vi "solar_voy_def Items Bit Offsets.vi"(10 "ITEMS in":T1[](array[typedef])) -> (1 "Bit Offsets":i32[](array[numeric]), 2 "ITEMS with Bit Offsets":T1[](array[typedef]))   [LabVIEW 2018]
doc: "This calculates the bit offsets for each item. If OFFSET is -1, this uses the current calculated bit offset."
uses:
  solar_voy_def_ctl ITEM TYPE.ctl
  type/solar_type Item Type.ctl
  solar_voy_def_ctl ITEM.ctl
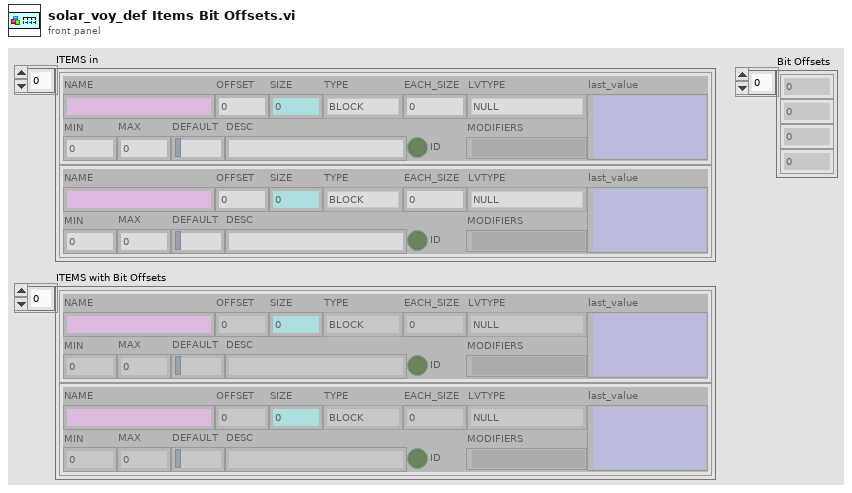
[diagram p1: front panel]
types:
  T1 = typedef "solar_voy_def_ctl ITEM.ctl" = cluster{"NAME":string, "OFFSET":i32, "SIZE":i32, "TYPE":T2, "EACH_SIZE":i32, "LVTYPE":T3, "MIN":dbl, "MAX":dbl, "DEFAULT":string, "DESC":string, "ID":bool, "MODIFIERS":variant, "last_value":variant}
  T2 = typedef "solar_voy_def_ctl ITEM TYPE.ctl" = enum8{"BLOCK", "INT", "UINT", "FLOAT", "STRING"}
  T3 = typedef "solar_type Item Type.ctl" = enum16{"NULL", "UNKNOWN", "CLUSTER", "I8", "I16", "I32", "I64", "U8", "U16", "U32", "U64", "U8_ENUM", "U16_ENUM", "U32_ENUM", "SGL", "DBL", "BOOLEAN", "STRING", "PATH", "VISA", "TAG", "TIME", "I8_1D", "I16_1D", "I32_1D", "I64_1D", "U8_1D", "U16_1D", "U32_1D", "U64_1D", "U8_ENUM_1D", "U16_ENUM_1D", "U32_ENUM_1D", "SGL_1D", "DBL_1D", "BOOLEAN_1D", "STRING_1D", "PATH_1D", "VISA_1D", "TAG_1D", "TIME_1D", "I8_2D", "I16_2D", "I32_2D", "I64_2D", "U8_2D", "U16_2D", "U32_2D", "U64_2D", "U8_ENUM_2D", "U16_ENUM_2D", "U32_ENUM_2D", "SGL_2D", "DBL_2D", "BOOLEAN_2D", "STRING_2D", "PATH_2D", "VISA_2D", "TAG_2D", "TIME_2D"}
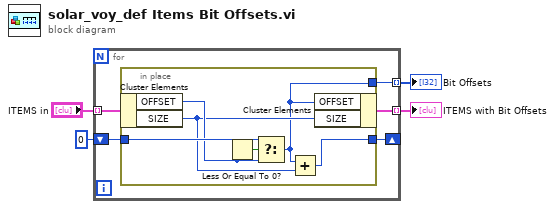
[diagram p0: block diagram]
diagram:
  n1 = for {
    tunnel: "ITEMS in" -> [w7] mode=indexing
    shift-right: [w8] -> _
    shift-left: 0 ("OFFSET") -> [w9]
    tunnel: [w6] -> w2 mode=indexing
    tunnel: [w5] -> w1 mode=indexing
    n2 = in-place {
      in-place-border: w9 -> [w15]
      in-place-border: [w13] -> w8
      in-place-border: [w10] -> w5
      n3 = in-place-cluster #1(w7) -> ("OFFSET"=w12:i32, "SIZE"=w11:i32)
      n4 = Less Or Equal To 0?(x=w12) -> (x <= 0?=w14:bool)
      n5 = Select(t=w15, s=w14, f=w12) -> (s? t:f=w10:i32)
      n6 = Add(x=w10, y=w11) -> (x+y=w13:i32)
      n7 = in-place-cluster #1("OFFSET"=w10, "SIZE"=w11) -> (w6:T1)
    }
  }
  "ITEMS with Bit Offsets" <- w2
  "Bit Offsets" <- w1
